vi "initialize_display.vi"() -> ()   [LabVIEW 2017]
uses:
  Downloads/ATM Simulator/Controls/DisplayControl.ctl
  controls/DisplayCommanda.ctl
  controls/EnableDisableCmd.ctl
  UpdateMessageControlla.ctl
  UpdateMessageCommanda.ctl
  controls/UpdateMenuCmd.ctl
  DisplayControl-czyjes.ctl
panel:
  out "queue out":refnum<queue>
  in  "queue":refnum<queue>
  out "error out":errorcluster
  in  "error in (no error)":errorcluster
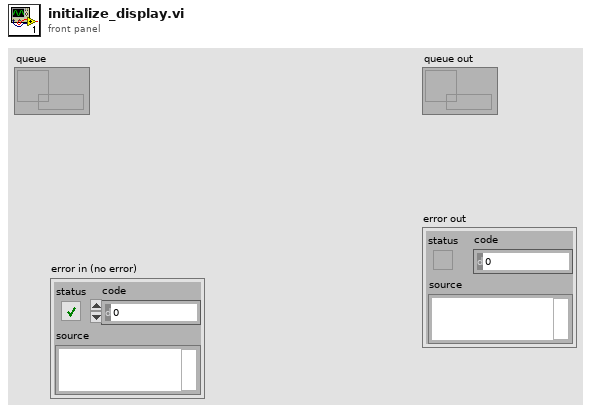
[diagram p1: front panel]
types:
  T1 = typedef "DisplayControl-czyjes.ctl" = cluster{"Command":T2, "Data":variant}
  T2 = typedef "DisplayCommanda.ctl" = enum16{"Initialize", "Enable/Disable Controls", "FocusCursor", "UpdateMessage", "UpdateMenus", "FinishOperation", "Exit", "CleanUserInput"}
  T3 = typedef "UpdateMenuCmd.ctl" = enum16{"NoMenu", "MainMenu"}
  T4 = typedef "UpdateMessageControlla.ctl" = cluster{"Command":T5, "Data":variant}
  T5 = typedef "UpdateMessageCommanda.ctl" = enum16{"Welcome", "MainMenu", "AccountFailed", "SessionTerminate", "Deposit", "DepositComplete", "Withdrawal", "WithdrawalComplete", "WithdrawalFailed", "BalanceInquiry"}
  T6 = typedef "EnableDisableCmd.ctl" = enum16{"InitialSetup", "Disable Menus", "Enable Menus", "Disable User Input", "Enable User Input"}
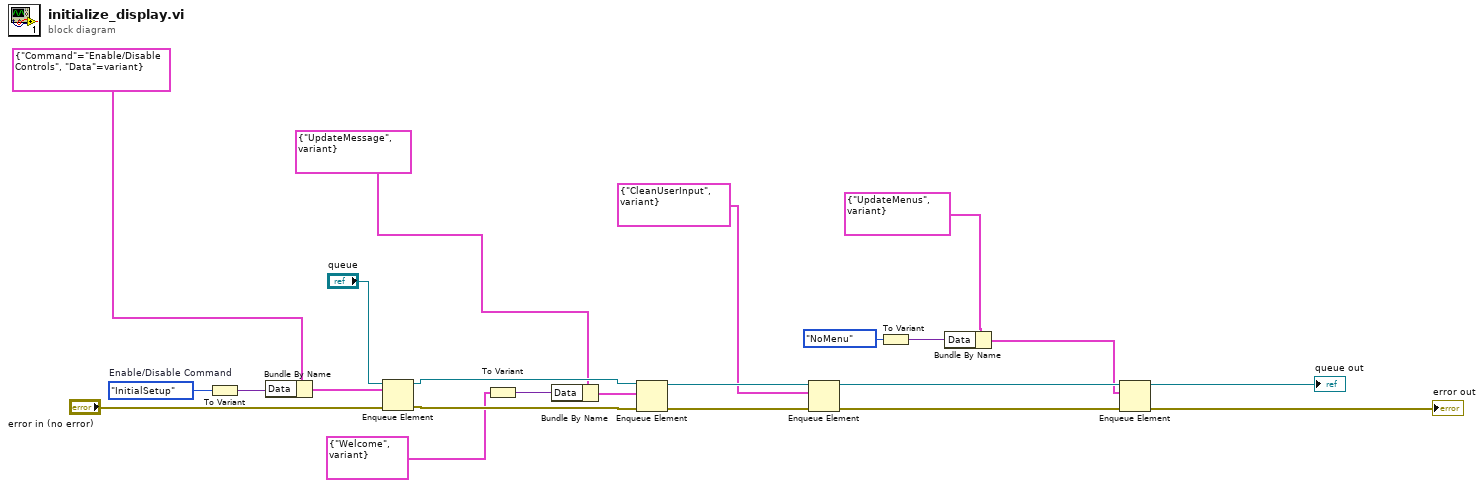
[diagram p0: block diagram]
diagram:
  w23 = EnableDisableCmd."InitialSetup"  # Enable/Disable Command
  n1 = To Variant(anything=w23) -> (Variant=w21:variant)
  n2 = Bundle By Name(cluster=T1 {"Command"=enum."Enable/Disable Controls", "Data"=variant} ("DisplayControl"), "Data"=w21) -> (w15:T1)
  n3 = Enqueue Element(queue="queue", element=w15, error in (no error)="error in (no error)") -> (queue out=w17:refnum<queue>, error out=w18:errorcluster)  [unwired: 1 in, 1 out]
  n4 = To Variant(anything=T4 {"Command"=enum."Welcome", "Data"=variant} ("UpdateMessageControl")) -> (Variant=w20:variant)
  n5 = Bundle By Name(cluster=T1 {"Command"=enum."UpdateMessage", "Data"=variant} ("DisplayControl"), "Data"=w20) -> (w19:T1)
  n6 = Enqueue Element(queue=w17, element=w19, error in (no error)=w18) -> (queue out=w13:refnum<queue>, error out=w12:errorcluster)  [unwired: 1 in, 1 out]
  n7 = Enqueue Element(queue=w13, element=T1 {"Command"=enum."CleanUserInput", "Data"=variant} ("DisplayControl"), error in (no error)=w12) -> (queue out=w11:refnum<queue>, error out=w10:errorcluster)  [unwired: 1 in, 1 out]
  n8 = To Variant(anything=UpdateMenuCmd."NoMenu" ("UpdateMenuCommand")) -> (Variant=w7:variant)
  n9 = Bundle By Name(cluster=T1 {"Command"=enum."UpdateMenus", "Data"=variant} ("DisplayControl"), "Data"=w7) -> (w1:T1)
  n10 = Enqueue Element(queue=w11, element=w1, error in (no error)=w10) -> (queue out=→"queue out":refnum<queue>, error out=→"error out":errorcluster)  [unwired: 1 in, 1 out]
